vi "Open All Relays_DAQmx_CreateTasks.vi"(0 "Device Name":string="Dev4", 1 "Physical Channels":string[](array[string])=["Dev1/port0", "Dev1/port1", "Dev1/port2"], 2 "initial value":u32, 3 "error in":errorcluster) -> (10 "error out":errorcluster)   [LabVIEW 2015]
uses:
  <vilib>/DAQmx/write.llb/DAQmx Write (Digital 1D U32 NChan 1Samp).vi
  <vilib>/DAQmx/miscellaneous.llb/DAQmx Fill In Error Info.vi
  <resource>/objmgr/daqmx.rc
panel:
  # "0 = OFF"
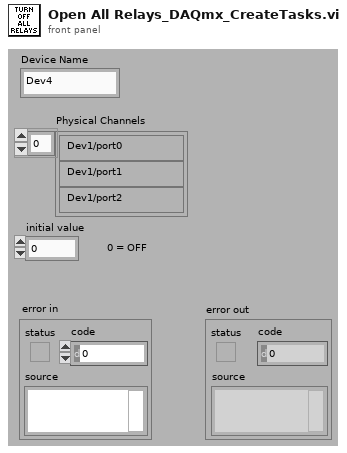
[diagram p1: front panel]
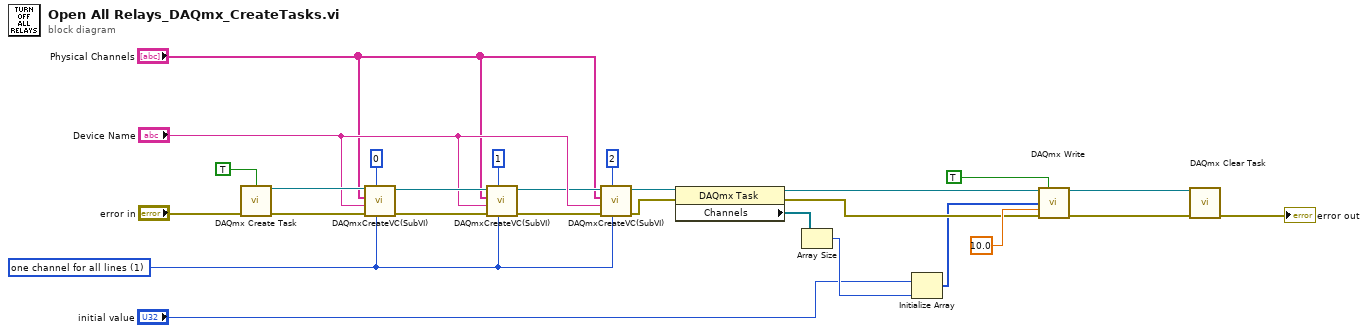
[diagram p0: block diagram]
diagram:
  w7 = 1 items=["one channel for each line", "one channel for all lines"] ("line grouping")
  n1 = call <vilib>:"DAQmx Create Task.vi"("auto cleanup"=TRUE, "error in"="error in") -> ("task out"=w24:refnum<k21>, "error out"=w25:errorcluster)  [unwired: 12 in]
  n2 = call "DAQmxCreateVC(SubVI).vi"("line grouping"=w7, "index"=0, "error in (no error)"=w25, "Device Name"="Device Name", "Physical Channels"="Physical Channels", "Refnum in"=w24) -> ("error out"=w10:errorcluster, "Refnum out"=w11:refnum<k21>)  [unwired: 3 in, 1 out]
  n3 = call "DAQmxCreateVC(SubVI).vi"("line grouping"=w7, "index"=1, "error in (no error)"=w10, "Device Name"="Device Name", "Physical Channels"="Physical Channels", "Refnum in"=w11) -> ("error out"=w3:errorcluster, "Refnum out"=w5:refnum<k21>)  [unwired: 3 in, 1 out]
  n4 = call "DAQmxCreateVC(SubVI).vi"("line grouping"=w7, "index"=2, "error in (no error)"=w3, "Device Name"="Device Name", "Physical Channels"="Physical Channels", "Refnum in"=w5) -> ("error out"=w2:errorcluster, "Refnum out"=w4:refnum<k21>)  [unwired: 3 in, 1 out]
  n5 = property class="DAQmx Task"(reference=w4, error in=w2) -> (reference out=w15:refnum<k21>, error out=w14:errorcluster, "Channels"=w16:refnum<k21>[])
  n6 = Array Size(array=w16) -> (size(s)=w18:i32)
  n7 = Initialize Array("initial value", w18) -> (w13:u32[])
  n8 = call-poly <vilib>:"DAQmx Write.vi"("task/channels in"=w15, "auto start"=TRUE, "data"=w13, "timeout"=10.0, "error in"=w14) -> ("task out"=w20:refnum<k21>, "error out"=w21:errorcluster)  [unwired: 8 in, 1 out]
  n9 = call <vilib>:"DAQmx Clear Task.vi"("task in"=w20, "error in"=w21) -> ("error out"=→"error out":errorcluster)  [unwired: 13 in]
